vi "Configure Stirrer Speed Setpoint.vi"(8 "error in (no error)":errorcluster, 10 "Stirrer Speed Setpoint":dbl min=0.0 max=1500.0, 11 "stirrer_interface in":refnum<class "stirrer_interface.lvclass">) -> (0 "error out":errorcluster, 3 "stirrer_interface out":refnum<class "stirrer_interface.lvclass">)   [LabVIEW 2020, in "polar_bear_plus_drivers.lvlib" / "stirrer_interface.lvclass"]
doc: "Configure the stirrer speed in range 0-1500 rpm. Minimum speed should be 200 rpm."
uses:
  <instrlib>/RxnRover/Driver Polar Bear Plus/stirrer_interface/stirrer_interface.lvclass
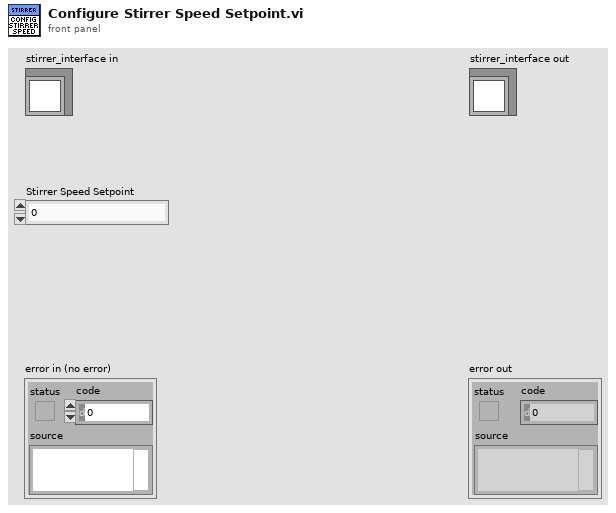
[diagram p1: front panel]
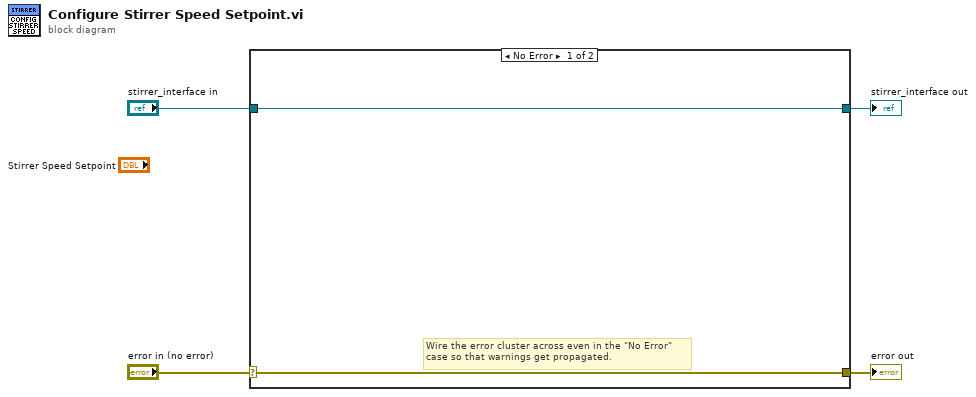
[diagram p0: block diagram]
diagram:
  n1 = case shown="No Error" "error in (no error)" {
    selector: "error in (no error)" -> [w5 w8]
    tunnel: [w5 w8] -> w3
    tunnel: [w6 w7] -> w1
    tunnel: "stirrer_interface in" -> [w6 w7]
    frame No Error {
      # "Wire the error cluster across even in the \"No Error\"\ncase so that warnings get propagated."
    }
    frame Error {
    }
  }
  "error out" <- w3
  "stirrer_interface out" <- w1
